vi "Start cRIO DAQ.vi"(8 "error in (no error)":errorcluster, 11 "cRIO IP":string="//172.22.11.2") -> (0 "error out":errorcluster, 5 "DAQ_AI_Reader endpoint":refnum<k21>, 7 "DAQ_CMD_Writer endpoint":refnum<k21>)   [LabVIEW 2024]
panel:
  in  "output cluster":T1
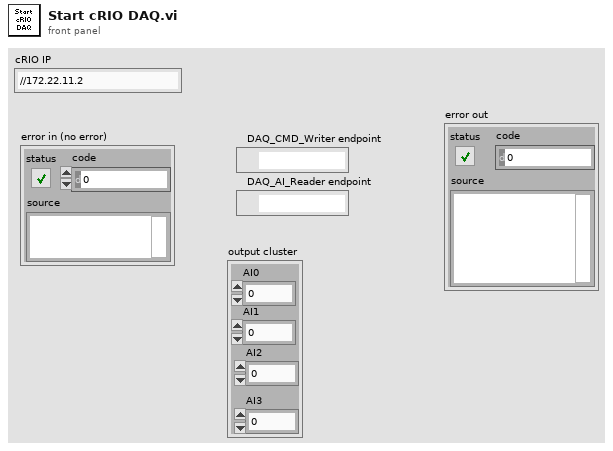
[diagram p1: front panel]
types:
  T1 = cluster{"AI0":dbl, "AI1":dbl, "AI2":dbl, "AI3":dbl}
  T2 = cluster{"Command":string, "Voltage":dbl, "Channel":string}
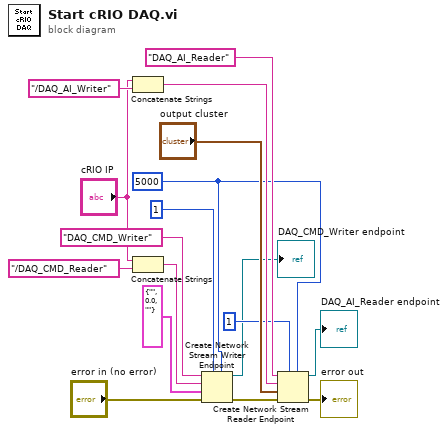
[diagram p0: block diagram]
diagram:
  w2 = 5000 ("timeout in ms (-1)")
  n1 = Concatenate Strings("cRIO IP", "/DAQ_AI_Writer" ("string")) -> (w9:string)
  n2 = Concatenate Strings("cRIO IP", "/DAQ_CMD_Reader" ("string")) -> (w13:string)
  n3 = Create Network Stream Writer Endpoint(5:w2, 7:1 ("writer buffer size"), 8:"error in (no error)", 9:T2 {"Command"="", "Voltage"=0.0, "Channel"=""} ("output cluster"), 10:w13, 11:"DAQ_CMD_Writer" ("writer name")) -> (0:w12:errorcluster, 3:→"DAQ_CMD_Writer endpoint":refnum<k21>)  [unwired: 1 in]
  n4 = Create Network Stream Reader Endpoint(5:w2, 7:1 ("reader buffer size"), 8:w12, 9:"output cluster", 10:w9, 11:"DAQ_AI_Reader" ("reader name")) -> (0:→"error out":errorcluster, 3:→"DAQ_AI_Reader endpoint":refnum<k21>)  [unwired: 1 in]
